vi "Read.vi"   [LabVIEW 2020, in "PICOTEST M351XA Series.lvlib"]
doc: "Reads and returns either single or multiple measurements from the instrument."
uses:
  PICOTEST M351XA Series.lvlib
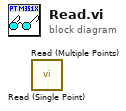
[diagram p0: block diagram]
diagram:
  n1 = call "Read (Single Point).vi"() -> ()  [unwired: 9 in, 3 out]
  n2 = call "Read (Multiple Points).vi"() -> ()  [unwired: 9 in, 3 out]
